vi "url_decode.vi"(11 "Message Body in":string) -> (3 "Message Body out":string)   [LabVIEW 2011]
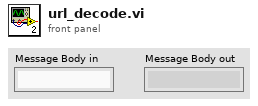
[diagram p1: front panel]
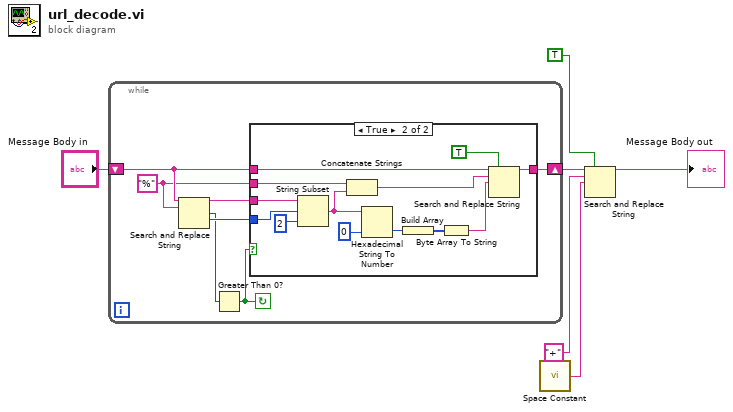
[diagram p0: block diagram]
diagram:
  n1 = while {
    shift-right: [w9] -> w5
    shift-left: "Message Body in" -> [w11]
    stop <- w7 continue-if-true
    w10 = "%" ("search string")
    n2 = Search and Replace String(input string=w11, search string=w10) -> (result string=w13:string, number of replacements=w8:i32, offset past replacement=w12:i32)  [unwired: 6 in, 1 out]
    n3 = Greater Than 0?(x=w8) -> (x > 0?=w7:bool)
    n4 = case shown="True" w7 {
      tunnel: w13 -> [_ w27]
      tunnel: w12 -> [_ w22]
      tunnel: w11 -> [w14 w21]
      tunnel: w10 -> [_ w20]
      tunnel: [w14 w15] -> w9
      frame False {
      }
      frame True {
        n5 = String Subset(string=w27, offset (0)=w22, length (rest)=2 ("length (rest)")) -> (substring=w18:string)
        n6 = Concatenate Strings(w20, w18) -> (w19:string)
        n7 = Hexadecimal String To Number(string=w18, default (0uL)=u8 0 ("default (0 U32)")) -> (number=w25:u8)  [unwired: 1 in, 1 out]
        n8 = Build Array(w25) -> (w24:u8[])
        n9 = Byte Array To String(unsigned byte array=w24) -> (string=w16:string)
        n10 = Search and Replace String(replace all?=TRUE ("replace all? (F)"), input string=w21, search string=w19, replace string=w16) -> (result string=w15:string)  [unwired: 4 in, 3 out]
      }
    }
  }
  n11 = call <vilib>:"Space Constant.vi"() -> ("String"=w1:string)
  n12 = Search and Replace String(replace all?=TRUE ("replace all? (F)"), input string=w5, search string="+", replace string=w1) -> (result string=→"Message Body out":string)  [unwired: 4 in, 3 out]
